vi "Generate IQ Waveform.vi"(2 "Selected Waveform":u16, 3 "Samples Per Cycle":i32=2 min=2 step=2) -> (0 "Q":dbl[](array[numeric]), 1 "I":dbl[](array[numeric]))   [LabVIEW 2021]
uses:
  <vilib>/Analysis/NI_AALBase.lvlib
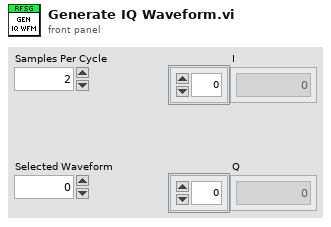
[diagram p1: front panel]
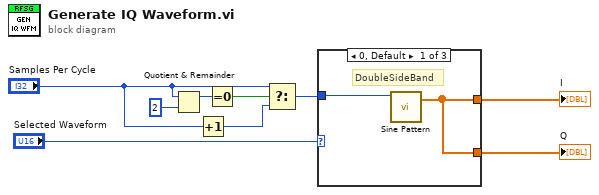
[diagram p0: block diagram]
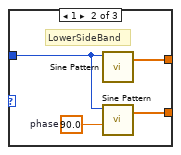
[diagram p2: hidden frame]
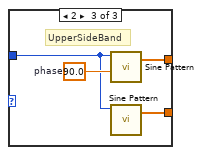
[diagram p3: hidden frame]
diagram:
  n1 = Quotient & Remainder(x="Samples Per Cycle", y=2) -> (x-y*floor(x/y)=w5:i32)  [unwired: 1 out]
  n2 = Increment(x="Samples Per Cycle") -> (x+1=w1:i32)
  n3 = Equal To 0?(x=w5) -> (x = 0?=w4:bool)
  n4 = Select(t="Samples Per Cycle", s=w4, f=w1) -> (s? t:f=w3:i32)
  n5 = case shown="0, Default" "Selected Waveform" {
    tunnel: [w11 w14 w19] -> w9
    tunnel: [w11 w13 w18] -> w8
    tunnel: w3 -> [w10 w12 w16]
    frame 0, Default {
      # "DoubleSideBand"
      n6 = call <vilib>:"Sine Pattern.vi"("samples"=w10) -> ("Sinusoidal Pattern"=w11:dbl[])  [unwired: 3 in, 1 out]
    }
    frame 1 {
      w15 = 90.0  # phase
      # "LowerSideBand"
      n7 = call <vilib>:"Sine Pattern.vi"("samples"=w12) -> ("Sinusoidal Pattern"=w14:dbl[])  [unwired: 3 in, 1 out]
      n8 = call <vilib>:"Sine Pattern.vi"("phase(degrees)"=w15, "samples"=w12) -> ("Sinusoidal Pattern"=w13:dbl[])  [unwired: 2 in, 1 out]
    }
    frame 2 {
      w17 = 90.0  # phase
      # "UpperSideBand"
      n9 = call <vilib>:"Sine Pattern.vi"("phase(degrees)"=w17, "samples"=w16) -> ("Sinusoidal Pattern"=w19:dbl[])  [unwired: 2 in, 1 out]
      n10 = call <vilib>:"Sine Pattern.vi"("samples"=w16) -> ("Sinusoidal Pattern"=w18:dbl[])  [unwired: 3 in, 1 out]
    }
  }
  "I" <- w9
  "Q" <- w8
